vi "Sub Initialize.vi"(8 "error in (no error)":errorcluster, 11 "Red Pitaya Digitizer in":refnum<class "Red Pitaya Digitizer.lvclass">) -> (0 "error out":errorcluster, 2 "Initialize Result":refnum<class "Acquired Result.lvclass">, 3 "Red Pitaya Digitizer out":refnum<class "Red Pitaya Digitizer.lvclass">)   [LabVIEW 2015, in "Red Pitaya Digitizer.lvclass"]
uses:
  Red Pitaya Digitizer.lvclass
  Results/Acquired Result/Acquired Result.lvclass
  Red Pitaya Digitizer.lvclass/Red Pitaya Digitizer.ctl
  NHMFL_Core/Libraries/Red Pitaya/RP Core/RP Instrument/RP Instrument.lvclass/RP Instrument.ctl
  Read RP Instrument.lvclass.vi
  NHMFL_Core/Libraries/Red Pitaya/RP Core/RP Instrument/Write Post-trigger samples.vi
  NHMFL_Core/Libraries/Red Pitaya/RP Core/RP Instrument/Write Decimation.vi
  Write RP Instrument.lvclass.vi
  Read RP Configuration.vi
  NHMFL_Core/Libraries/Red Pitaya/RP Core/RP Instrument/RP Instrument.lvclass
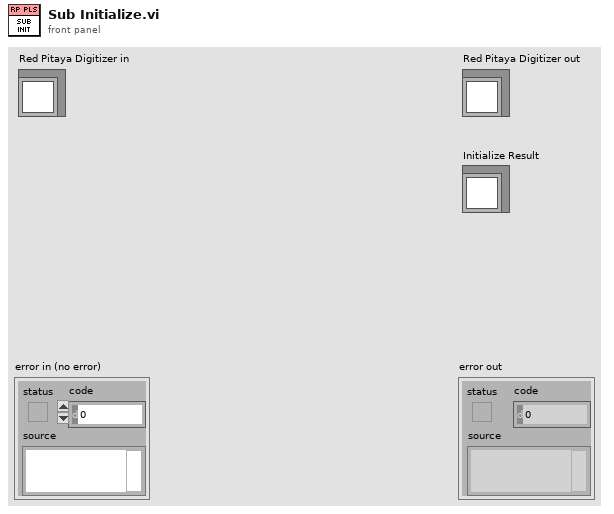
[diagram p1: front panel]
types:
  T1 = typedef "RP Configuration.ctl" = cluster{"Ranges":dbl[], "Output frequency 1":dbl, "Output frequency 2":dbl, "Pre-trigger samples":i32, "Post-trigger samples":u64, "Desimation rate":u64, "Delayed start":u64}
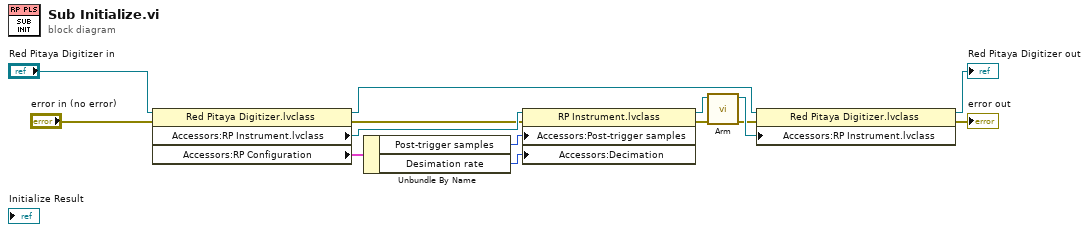
[diagram p0: block diagram]
diagram:
  n1 = property class="Red Pitaya Digitizer.lvclass"(reference="Red Pitaya Digitizer in", error in="error in (no error)") -> (reference out=w5:refnum<class "Red Pitaya Digitizer.lvclass">, error out=w6:errorcluster, "Accessors:RP Instrument.lvclass"=w13:refnum<class "RP Instrument.lvclass">, "Accessors:RP Configuration"=w11:T1)
  n2 = Unbundle By Name(w11) -> ("Post-trigger samples"=w10:u64, "Desimation rate"=w9:u64)
  n3 = property class="RP Instrument.lvclass"(reference=w13, error in=w6, "Accessors:Post-trigger samples"=w10, "Accessors:Decimation"=w9) -> (reference out=w12:refnum<class "RP Instrument.lvclass">, error out=w7:errorcluster)
  n4 = call-dynamic "Arm.vi"("error in (no error)"=w7, "RP Instrument in"=w12) -> ("error out"=w2:errorcluster, "RP Instrument out"=w3:refnum<class "RP Instrument.lvclass">)  [unwired: 8 in]
  n5 = property class="Red Pitaya Digitizer.lvclass"(reference=w5, error in=w2, "Accessors:RP Instrument.lvclass"=w3) -> (reference out=→"Red Pitaya Digitizer out":refnum<class "Red Pitaya Digitizer.lvclass">, error out=→"error out":errorcluster)
